vi "Initiate Autocal.vi"(8 "error in":errorcluster, 10 "mode (ALL)":T1, 11 "VISA resource in":refnum<visa-resource-name>) -> (0 "error out":errorcluster, 3 "VISA resource out":refnum<visa-resource-name>)   [LabVIEW 2018, in "3458A Virtual Digitizer.lvlib" / "3458A Digitizing Low Levels.lvlib"]
doc: "Initiates auto-calibration routine. Does not wait for finish. Use 'Wait for Device Ready' to detect end of calibration.\n\nNote: Reentrant VI so it can be executed in parallel for multiple 3458A sessions."
uses:
  3458A Digitizing Low Levels.lvlib
  AutoCal Mode.ctl
  3458A Basic Driver/3458A Basic Driver.lvlib
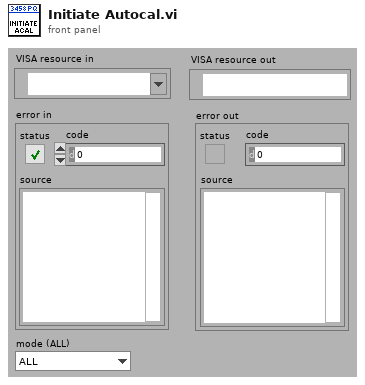
[diagram p1: front panel]
types:
  T1 = typedef "3458A Virtual Digitizer.lvlib/3458A Digitizing Low Levels.lvlib/AutoCal Mode.ctl" = enum16{"ALL", "DCV", "AC", "OHMS"}
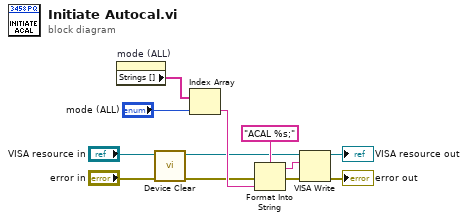
[diagram p0: block diagram]
diagram:
  n1 = property on="mode (ALL)" class="Enum (strict)"() -> ("Strings []"=w6:string[])  [unwired: 2 in, 2 out]
  n2 = call "Device Clear.vi"("error in(no error)"="error in", "VISA Resource Name"="VISA resource in") -> ("error out"=w3:errorcluster, "VISA resource name out"=w2:refnum<visa-resource-name>)  [unwired: 8 in]
  n3 = Index Array(array=w6, index="mode (ALL)") -> (element=w5:string)
  n4 = Format Into String(format string="ACAL %s;" ("write buffer"), error in=w3, w5) -> (resulting string=w8:string, error out=w10:errorcluster)  [unwired: 1 in]
  n5 = VISA Write(VISA resource name=w2, write buffer=w8, error in (no error)=w10) -> (VISA resource name out=→"VISA resource out":refnum<visa-resource-name>, error out=→"error out":errorcluster)  [unwired: 1 out]
